vi "Exemple_Extraction_DictVectorizer.vi"() -> ()   [LabVIEW 2020]
uses:
  Objet/6 - Datasets Transformation/6.2 - Feature extraction/DictVectorizer/DictVectorizer.lvclass
panel:
  in  "X":cluster{"Key":string[], "Value":i32[]}={"Key"=["foo", "bar", "foo", "baz"], "Value"=[1, 2, 3, 1]}
  in  "DictVectorizer":T1={"dtype"="float", "separator"="=", "sparse"=TRUE, "sort"=TRUE}
  out "Data":T2
  out "error out":errorcluster caption="sortie d'erreur"
  in  "error in":errorcluster caption="entrée d'erreur"
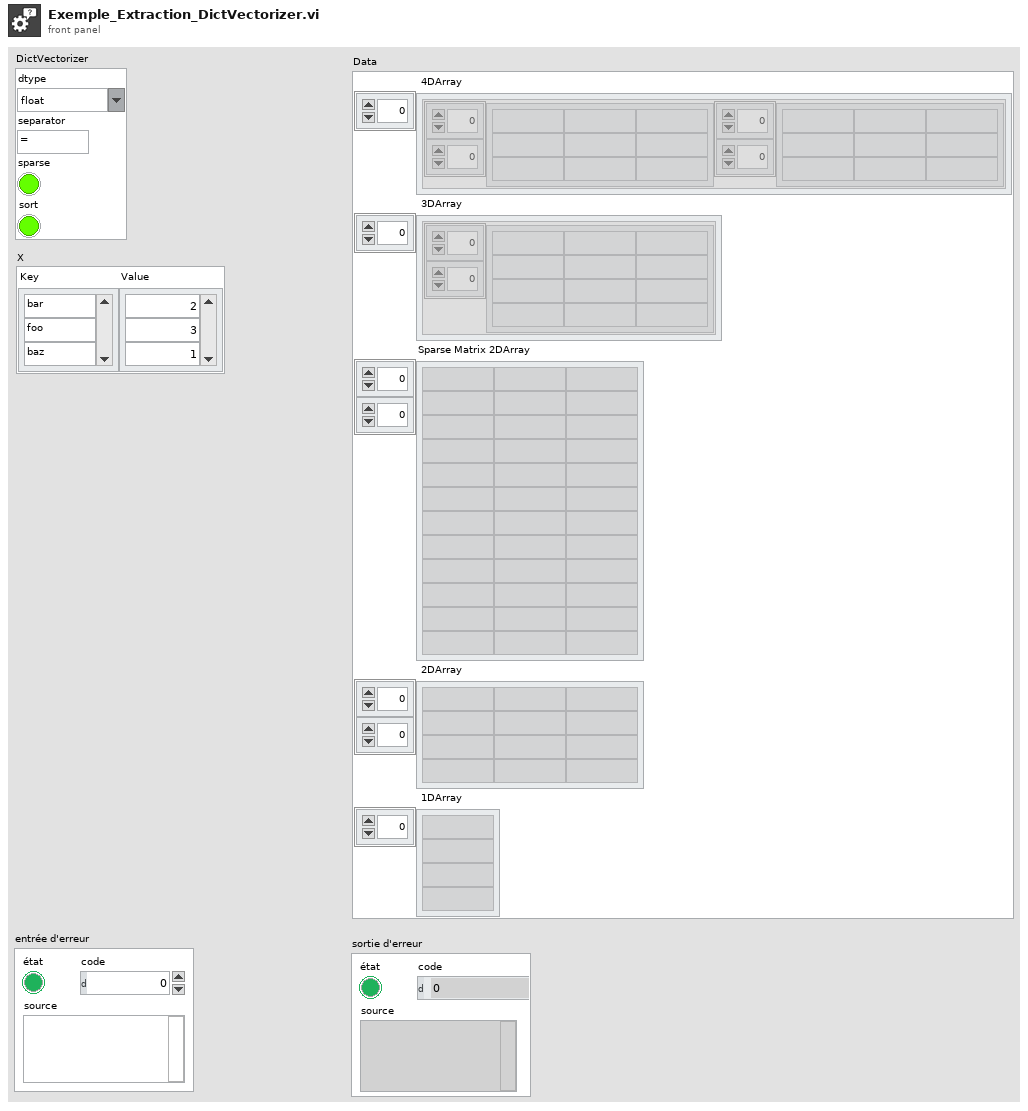
[diagram p1: front panel]
types:
  T1 = cluster{"dtype":string, "separator":string, "sparse":bool, "sort":bool}
  T2 = cluster{" 4DArray":cluster{"1":string[][], "2":string[][]}[], " 3DArray":cluster{"Tableau":string[][]}[], "Sparse Matrix 2DArray":string[][], " 2DArray":string[][], " 1DArray":string[]}
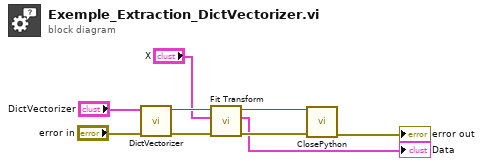
[diagram p0: block diagram]
diagram:
  n1 = call "DictVectorizer.vi"("error in"="error in", "DictVectorizer"="DictVectorizer") -> ("error out"=w6:errorcluster, "DictVectorizer.lvclass"=w7:refnum<class "DictVectorizer.lvclass">)  [unwired: 8 in]
  n2 = call-dynamic "Fit Transform.vi"("error in (no error)"=w6, "X"="X", "DictVectorizer.lvclass"=w7) -> ("error out"=w4:errorcluster, "Data"=→"Data":T2, "DictVectorizer.lvclass"=w5:refnum<class "DictVectorizer.lvclass">)  [unwired: 6 in]
  n3 = call-dynamic "ClosePython.vi"("error in (no error)"=w4, "Scikit-learn en entrée"=w5) -> ("error out"=→"error out":errorcluster)  [unwired: 8 in, 1 out]
